vi "Validate.vi"(3 "message":string) -> (0 "Ok":bool, 1 "End":bool)   [LabVIEW 2019]
panel:
  in  "Cancel Button":bool
  in  "OK Button":bool
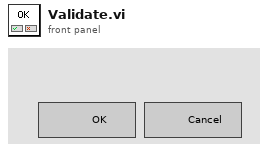
[diagram p1: front panel]
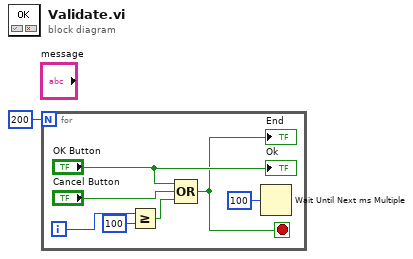
[diagram p0: block diagram]
diagram:
  n1 = for {
    N: 200 -> [_]
    i -> [w2]
    stop <- w3 stop-if-true
    n2 = Greater Or Equal?(x=w2, y=100) -> (x >= y?=w8:bool)
    n3 = Compound Arithmetic op=OR("OK Button", "Cancel Button", w8) -> (w3:bool)
    "End" <- w3
    n4 = Wait Until Next ms Multiple(millisecond multiple=u32 100) -> ()  [unwired: 1 out]
    "Ok" <- "OK Button"
  }
